vi "Twist3d_Equals.vi"(9 "other Twist3d":T1, 11 "this Twist3d":T1) -> (3 "Equals":bool)   [LabVIEW 2019, in "Trajectory_Library.lvlib"]
doc: "Checks equality between this Twist3d and another Twist3d.\n\nParameters:\n - this twist3d -- This TWIST data structure\n - other twist3d -- The other TWIST data structure to compare to\n\nReturns:\n - equals - Returns TRUE if both TWISTS are equal"
uses:
  Trajectory_Library.lvlib
  TypeDef/TWIST3D.ctl
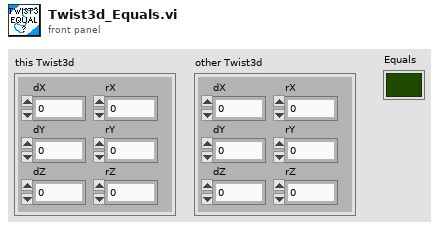
[diagram p1: front panel]
types:
  T1 = typedef "Trajectory_Library.lvlib/TWIST3D.ctl" = cluster{"dX":dbl, "dY":dbl, "dZ":dbl, "rX":dbl, "rY":dbl, "rZ":dbl}
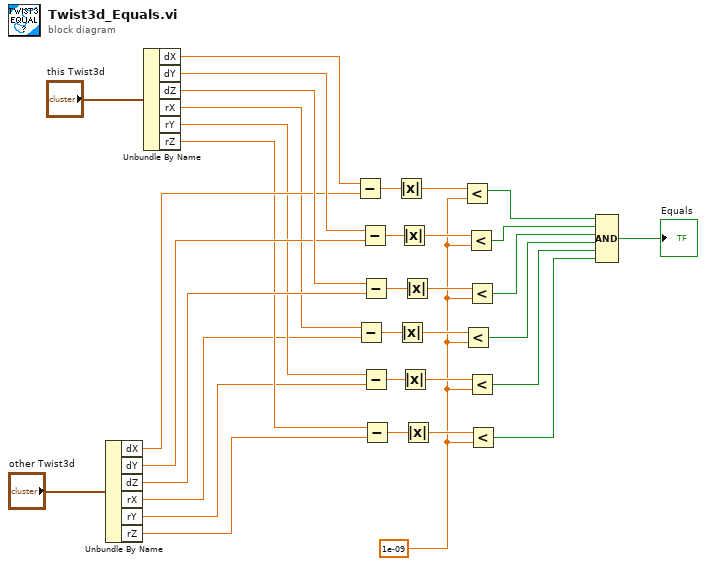
[diagram p0: block diagram]
diagram:
  w10 = 1e-09 ("y")
  n1 = Unbundle By Name("other Twist3d") -> ("dX"=w19:dbl, "dY"=w18:dbl, "dZ"=w17:dbl, "rX"=w3:dbl, "rY"=w2:dbl, "rZ"=w1:dbl)
  n2 = Unbundle By Name("this Twist3d") -> ("dX"=w22:dbl, "dY"=w21:dbl, "dZ"=w20:dbl, "rX"=w6:dbl, "rY"=w5:dbl, "rZ"=w4:dbl)
  n3 = Subtract(x=w22, y=w19) -> (x-y=w25:dbl)
  n4 = Subtract(x=w6, y=w3) -> (x-y=w13:dbl)
  n5 = Subtract(x=w21, y=w18) -> (x-y=w24:dbl)
  n6 = Subtract(x=w20, y=w17) -> (x-y=w23:dbl)
  n7 = Subtract(x=w5, y=w2) -> (x-y=w12:dbl)
  n8 = Subtract(x=w4, y=w1) -> (x-y=w11:dbl)
  n9 = Absolute Value(x=w25) -> (abs(x)=w28:dbl)
  n10 = Absolute Value(x=w13) -> (abs(x)=w16:dbl)
  n11 = Absolute Value(x=w24) -> (abs(x)=w27:dbl)
  n12 = Absolute Value(x=w12) -> (abs(x)=w15:dbl)
  n13 = Absolute Value(x=w23) -> (abs(x)=w26:dbl)
  n14 = Absolute Value(x=w11) -> (abs(x)=w14:dbl)
  n15 = Less?(x=w28, y=w10) -> (x < y?=w32:bool)
  n16 = Less?(x=w16, y=w10) -> (x < y?=w9:bool)
  n17 = Less?(x=w27, y=w10) -> (x < y?=w31:bool)
  n18 = Less?(x=w26, y=w10) -> (x < y?=w30:bool)
  n19 = Less?(x=w15, y=w10) -> (x < y?=w8:bool)
  n20 = Less?(x=w14, y=w10) -> (x < y?=w7:bool)
  n21 = Compound Arithmetic op=AND(w32, w31, w30, w9, w8, w7) -> (→"Equals":bool)
